vi "NewLogFile.vi"(8 "error in (no error)":errorcluster, 11 "S4GUI in":refnum<class "S4GUI.lvclass">) -> (0 "error out":errorcluster, 3 "S4GUI out":refnum<class "S4GUI.lvclass">)   [LabVIEW 2018, in "S4GUI.lvclass"]
uses:
  S4GUI.lvclass
  S4GUI.lvclass/S4GUI.ctl
  Log/Log.lvclass
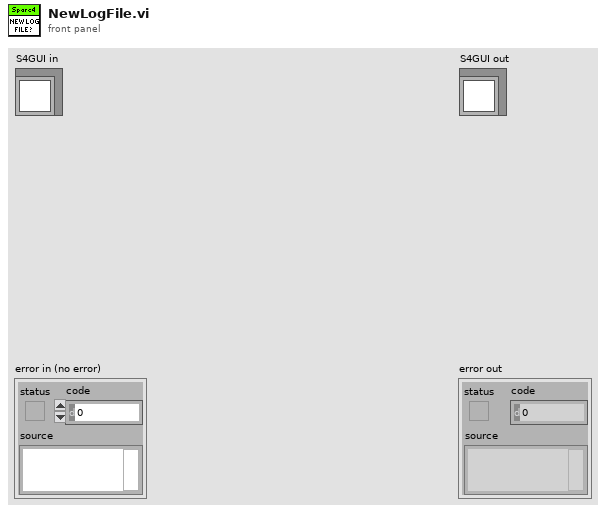
[diagram p1: front panel]
types:
  T1 = enum16{"open", "replace", "create", "open or create", "replace or create", "replace or create with confirmation"}
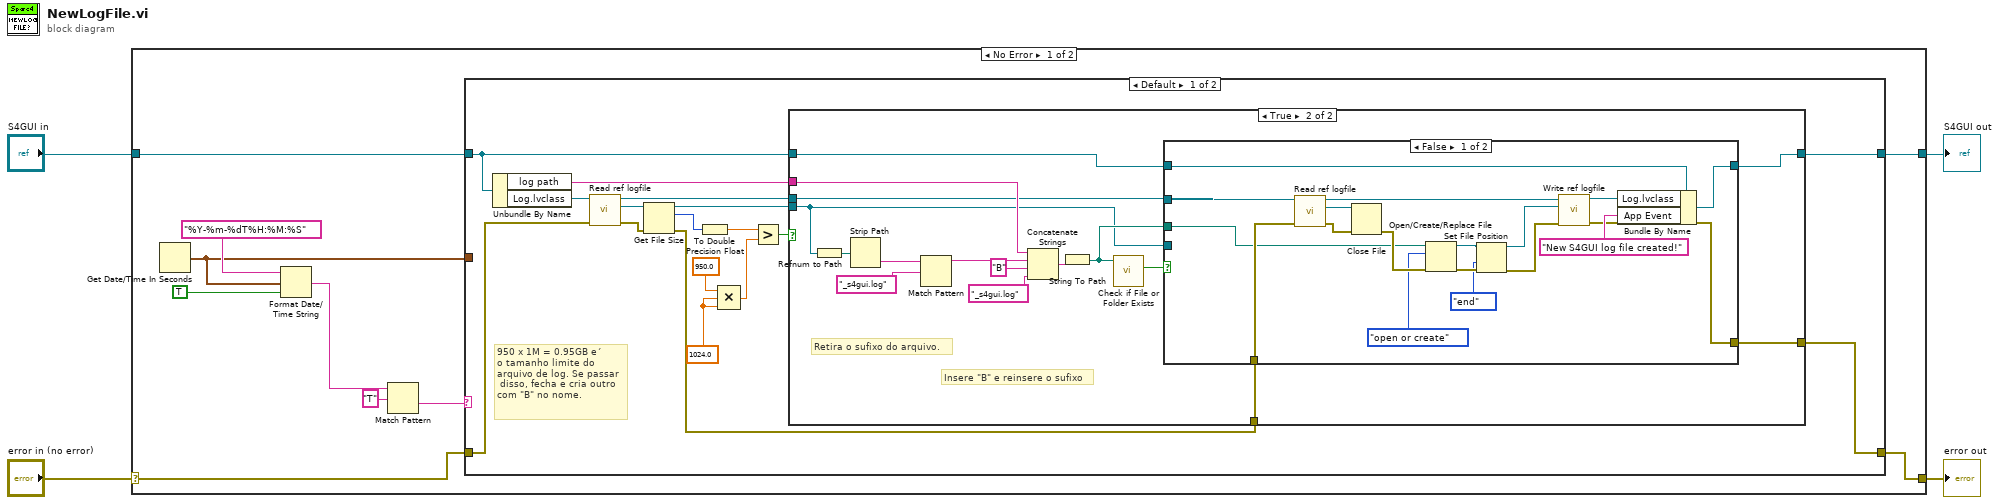
[diagram p0: block diagram]
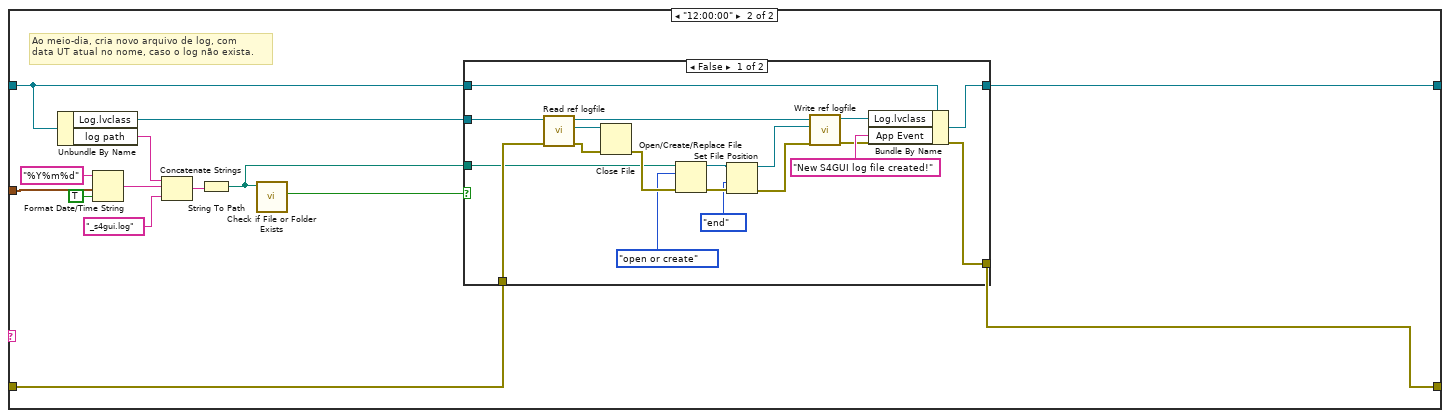
[diagram p4: hidden frame]
diagram:
  n1 = case shown="No Error" "error in (no error)" {
    selector: "error in (no error)" -> [w7 w105]
    tunnel: [w6 w105] -> w3
    tunnel: [w8 w104] -> w1
    tunnel: "S4GUI in" -> [w9 w104]
    frame No Error {
      n2 = Get Date/Time In Seconds() -> (seconds since 1Jan1904=w5:timestamp)
      n3 = Format Date/Time String(time format string (%c)="%Y-%m-%dT%H:%M:%S", seconds (now)=w5, UTC format=TRUE) -> (date/time string=w12:string)
      n4 = Match Pattern(string=w12, regular expression="T") -> (after substring=w10:string)  [unwired: 1 in, 3 out]
      n5 = case shown="Default" w10 {
        tunnel: [w21 w70] -> w8
        tunnel: w9 -> [w22 w71]
        tunnel: w7 -> [w18 w77]
        tunnel: [w19 w73] -> w6
        tunnel: w5 -> [_ w82]
        frame Default {
          w15 = 1024.0 ("y")
          # "950 x 1M = 0.95GB e´\no tamanho limite do \narquivo de log. Se passar\n disso, fecha e cria outro \ncom \"B\" no nome."
          n6 = Unbundle By Name(w22) -> ("log path"=w24:string, "Log.lvclass"=w31:refnum<class "Log.lvclass">)
          n7 = call-dynamic "Read ref logfile.vi"("error in (no error)"=w18, "Log in"=w31) -> ("error out"=w17:errorcluster, "ref logfile"=w30:refnum<file>, "Log out"=w23:refnum<class "Log.lvclass">)  [unwired: 7 in]
          n8 = Get File Size(file=w30, error in=w17) -> (refnum out=w20:refnum<file>, size (in bytes)=w27:i64, 0:w16:errorcluster)
          n9 = To Double Precision Float(number=w27) -> (double precision float=w26:dbl)
          n10 = Compound Arithmetic op=MULTIPLY(950.0 ("value"), w15, w15) -> (w28:dbl)
          n11 = Greater?(x=w26, y=w28) -> (0:w25:bool)
          n12 = case shown="True" w25 {
            tunnel: w24 -> [_ w47]
            tunnel: w23 -> [_ w44]
            tunnel: w22 -> [w33 w43]
            tunnel: [w33 w42] -> w21
            tunnel: w16 -> [w32 w41]
            tunnel: w20 -> [_ w38]
            tunnel: [w32 w39] -> w19
            frame False {
            }
            frame True {
              # "Insere \"B\" e reinsere o sufixo"
              # "Retira o sufixo do arquivo."
              n13 = Refnum to Path(1:w38) -> (0:w37:path)
              n14 = Strip Path(path=w37) -> (name=w36:string)  [unwired: 1 out]
              n15 = Match Pattern(string=w36, regular expression="_s4gui.log" ("string")) -> (before substring=w34:string)  [unwired: 1 in, 3 out]
              n16 = Concatenate Strings(w47, w34, "B" ("string"), "_s4gui.log" ("string")) -> (w48:string)
              n17 = String To Path(string=w48) -> (path=w40:path)
              n18 = call <vilib>:"Check if File or Folder Exists.vi"("path"=w40) -> ("file or folder exists?"=w45:bool)  [unwired: 8 in, 2 out]
              n19 = case shown="False" w45 {
                tunnel: w44 -> [w67 _]
                tunnel: w41 -> [w66 w69]
                tunnel: [w51 w69] -> w39
                tunnel: w38 -> [_ _]
                tunnel: [w53 w68] -> w42
                tunnel: w43 -> [w58 w68]
                tunnel: w40 -> [w50 _]
                frame False {
                  n20 = call-dynamic "Read ref logfile.vi"("error in (no error)"=w66, "Log in"=w67) -> ("error out"=w64:errorcluster, "ref logfile"=w65:refnum<file>, "Log out"=w56:refnum<class "Log.lvclass">)  [unwired: 7 in]
                  n21 = Close File(refnum=w65, error in=w64) -> (error out=w63:errorcluster)  [unwired: 1 out]
                  n22 = Open/Create/Replace File(file path (use dialog)=w50, error in=w63, operation (0:open)=T1."open or create") -> (refnum out=w59:refnum<file>, error out=w61:errorcluster)  [unwired: 3 in, 1 out]
                  n23 = Set File Position(refnum=w59, from (0:start)=enum16{"start", "end", "current"}."end", error in=w61) -> (refnum out=w57:refnum<file>, error out=w52:errorcluster)  [unwired: 1 in]
                  n24 = call-dynamic "Write ref logfile.vi"("error in (no error)"=w52, "ref logfile"=w57, "Log in"=w56) -> ("error out"=w51:errorcluster, "Log out"=w55:refnum<class "Log.lvclass">)  [unwired: 7 in]
                  n25 = Bundle By Name(cluster=w58, "Log.lvclass"=w55, "App Event"="New S4GUI log file created!") -> (w53:refnum<class "S4GUI.lvclass">)
                }
                frame True {
                }
              }
            }
          }
        }
        frame "12:00:00" {
          # "Ao meio-dia, cria novo arquivo de log, com\ndata UT atual no nome, caso o log não exista."
          n26 = Unbundle By Name(w71) -> ("Log.lvclass"=w78:refnum<class "Log.lvclass">, "log path"=w76:string)
          n27 = Format Date/Time String(time format string (%c)="%Y%m%d", seconds (now)=w82, UTC format=TRUE) -> (date/time string=w80:string)
          n28 = Concatenate Strings(w76, w80, "_s4gui.log" ("string")) -> (w75:string)
          n29 = String To Path(string=w75) -> (path=w72:path)
          n30 = call <vilib>:"Check if File or Folder Exists.vi"("path"=w72) -> ("file or folder exists?"=w74:bool)  [unwired: 8 in, 2 out]
          n31 = case shown="False" w74 {
            tunnel: w78 -> [w101 _]
            tunnel: w77 -> [w100 w103]
            tunnel: [w84 w103] -> w73
            tunnel: w72 -> [w96 _]
            tunnel: [w86 w102] -> w70
            tunnel: w71 -> [w91 w102]
            frame False {
              n32 = call-dynamic "Read ref logfile.vi"("error in (no error)"=w100, "Log in"=w101) -> ("error out"=w98:errorcluster, "ref logfile"=w99:refnum<file>, "Log out"=w89:refnum<class "Log.lvclass">)  [unwired: 7 in]
              n33 = Close File(refnum=w99, error in=w98) -> (error out=w97:errorcluster)  [unwired: 1 out]
              n34 = Open/Create/Replace File(file path (use dialog)=w96, error in=w97, operation (0:open)=T1."open or create") -> (refnum out=w92:refnum<file>, error out=w94:errorcluster)  [unwired: 3 in, 1 out]
              n35 = Set File Position(refnum=w92, from (0:start)=enum16{"start", "end", "current"}."end", error in=w94) -> (refnum out=w90:refnum<file>, error out=w85:errorcluster)  [unwired: 1 in]
              n36 = call-dynamic "Write ref logfile.vi"("error in (no error)"=w85, "ref logfile"=w90, "Log in"=w89) -> ("error out"=w84:errorcluster, "Log out"=w88:refnum<class "Log.lvclass">)  [unwired: 7 in]
              n37 = Bundle By Name(cluster=w91, "Log.lvclass"=w88, "App Event"="New S4GUI log file created!") -> (w86:refnum<class "S4GUI.lvclass">)
            }
            frame True {
            }
          }
        }
      }
    }
    frame Error {
    }
  }
  "error out" <- w3
  "S4GUI out" <- w1
